vi "get runtime class name.vi"(8 "error in":errorcluster, 11 "engine configuration in":refnum<class "engine configuration.lvclass">) -> (0 "error out":errorcluster, 2 "class name":string, 3 "engine configuration out":refnum<class "engine configuration.lvclass">)   [LabVIEW 2013, in "engine configuration.lvclass"]
doc: "This property is used to find the name of the runtime class that accepts the configuration class as an input to its initialize function. This linkage is done to prevent a hard dependency between the two objects which would prevent the configuration object from being OS agnostic."
uses:
  engine configuration.lvclass
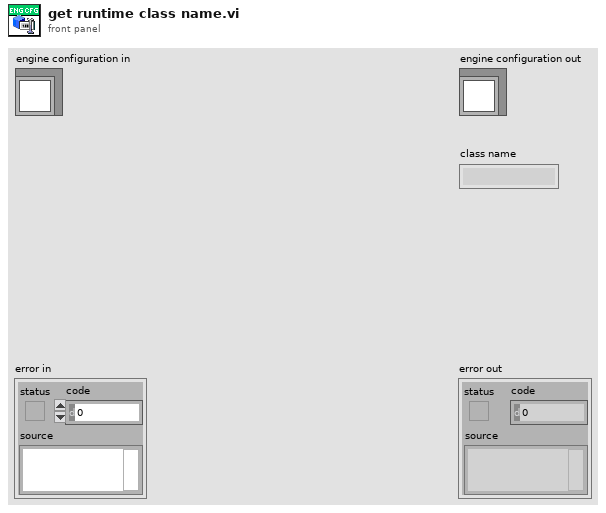
[diagram p1: front panel]
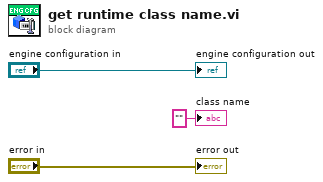
[diagram p0: block diagram]
diagram:
  "error out" <- "error in"
  "engine configuration out" <- "engine configuration in"
  "class name" <- "" ("class name")
